vi "LCD Create Custom Char.vi"(0 "Arduino Resource":T3, 5 "Custom Char Number":u8, 7 "LCD Character":T1, 11 "error in":errorcluster) -> (4 "Arduino Resource":T3, 15 "error":errorcluster)   [LabVIEW 2015, in "LabVIEW Interface for Arduino.lvlib"]
doc: "Creates a custom character, which can be later printed on the LCD screen. This function supports 5x8 pixels. Note, after creating a new character the LCD screen must be reinitilized using the LCD Init VI. Also, the custom character can be printed using the LCD Print Custom Char VI."
uses:
  <vilib>/LabVIEW Interface for Arduino/LabVIEW Interface for Arduino.lvlib
  <vilib>/LabVIEW Interface for Arduino/Type Defs/Arduino Resource.ctl
  <vilib>/LabVIEW Interface for Arduino/Type Defs/Board Type.ctl
  <vilib>/LabVIEW Interface for Arduino/Type Defs/LCD Character.ctl
  <vilib>/LabVIEW Interface for Arduino/Type Defs/LCD Char Row.ctl
  <vilib>/LabVIEW Interface for Arduino/Type Defs/Command.ctl
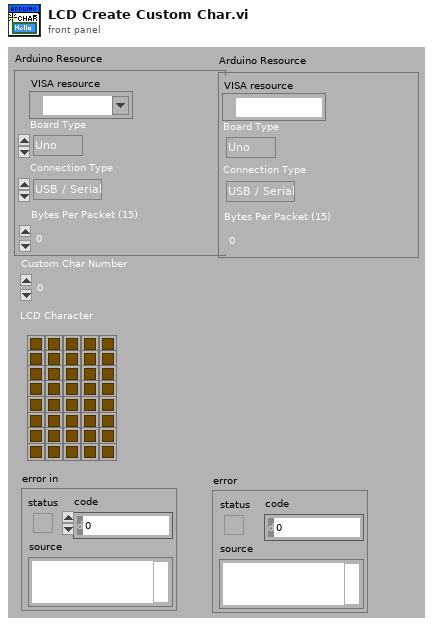
[diagram p1: front panel]
types:
  T1 = typedef "LabVIEW Interface for Arduino.lvlib/LCD Character.ctl" = cluster{"Row 0":T2, "Row 1":T2, "Row 2":T2, "Row 3":T2, "Row 4":T2, "Row 5":T2, "Row 6":T2, "Row 7":T2}
  T2 = typedef "LabVIEW Interface for Arduino.lvlib/LCD Char Row.ctl" = cluster{"LED 4":bool, "LED 3":bool, "LED 2":bool, "LED 1":bool, "LED 0":bool}
  T3 = typedef "LabVIEW Interface for Arduino.lvlib/Arduino Resource.ctl" = cluster{"VISA resource":refnum<visa-resource-name>, "Board Type":T4, "Connection Type":enum8{"USB / Serial"}, "Bytes Per Packet (15)":u8}
  T4 = typedef "LabVIEW Interface for Arduino.lvlib/Board Type.ctl" = enum16{"Uno", "Dimuelanove w/Atmega 328", "Mega 2560"}
  T5 = typedef "LabVIEW Interface for Arduino.lvlib/Command.ctl" = enum8{"setArduinoMode", "flushSerial", "setPinMode", "digitalWritePin", "digitalWritePort", "tone", "digitalReadPin", "digitalReadPort", "analogReadPin", "analogReadPort", "pwmWritePin", "pwmWritePort", "sevenSegment_Configure", "sevenSegment_Write", "I2C Init", "I2C Write", "I2C Read", "SPI Init", "SPI Set Bit Order", "SPI Set Clock Divider", "SPI Set Data Mode", "SPI Send / Receive", "SPI Close", "Servo Set Num Servos", "Servo Config Servo", "Servo Write Angle", "Servo Read Angle", "Servo Write Pulse Width", "Servo Read Pulse Width", "Servo Detach", "LCD Init", "LCD Set Size", "LCD Set Cursor Mode", "LCD Clear", "LCD Set Cursor Position", "LCD Print", "LCD Display Power", "LCD Scroll Display", "LCD Autoscroll", "LCD Print Direction", "LCD Create Custom Char", "LCD Print Custom Char", "contAcqOn", "contAcqOff", "getFirmwareVersion", "FiniteSampleStart"}
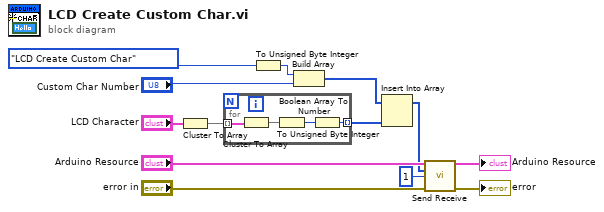
[diagram p0: block diagram]
diagram:
  n1 = Cluster To Array(cluster="LCD Character") -> (array=w5:T2[])
  n2 = for {
    tunnel: w5 -> [w17] mode=indexing
    tunnel: [w14] -> w4 mode=indexing
    n3 = Cluster To Array(cluster=w17) -> (array=w16:bool[])
    n4 = Boolean Array To Number(Boolean array=w16) -> (number=w15:u32)
    n5 = To Unsigned Byte Integer(number=w15) -> (unsigned 8bit integer=w14:u8)
  }
  n6 = To Unsigned Byte Integer(number=Command."LCD Create Custom Char" ("Command")) -> (unsigned 8bit integer=w12:u8)
  n7 = Build Array(w12, "Custom Char Number") -> (w3:u8[])
  n8 = Insert Into Array(array=w3, new element=w4) -> (w2:u8[])  [unwired: 1 in]
  n9 = call <vilib>:"Send Receive.vi"("Arduino Resource"="Arduino Resource", "Data"=w2, "Bytes To Read (0)"=u8 1, "error in"="error in") -> ("Arduino Resource"=→"Arduino Resource":T3, "error out"=→"error":errorcluster)  [unwired: 9 in, 1 out]
